vi "RFConfig_SubVI_HMCT22##_PowerOnOff.vi"(8 "error in (no error)":errorcluster, 9 "Power On?":bool, 10 "Boolean in":bool, 11 "VISA Refnum in":refnum<visa-resource-name>) -> (0 "error out":errorcluster, 3 "Boolean out":bool)   [LabVIEW 2019]
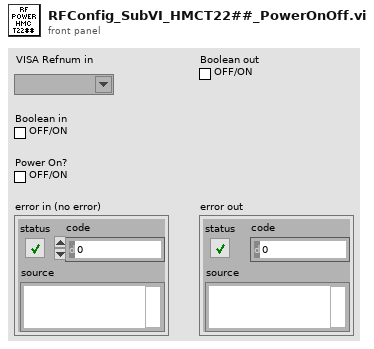
[diagram p1: front panel]
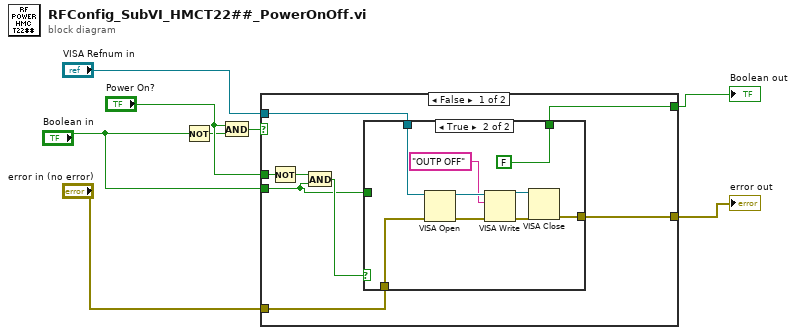
[diagram p0: block diagram]
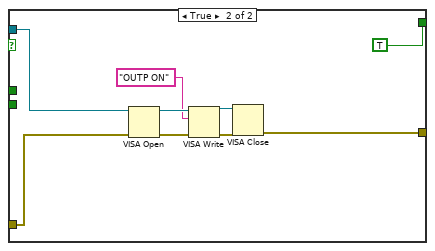
[diagram p3: hidden frame]
diagram:
  n1 = Not(x="Boolean in") -> (.not. x?=w4:bool)
  n2 = And(x="Power On?", y=w4) -> (x .and. y?=w1:bool)
  n3 = case shown="False" w1 {
    tunnel: [w11 w29] -> w2
    tunnel: "error in (no error)" -> [w12 w35]
    tunnel: "Power On?" -> [w15 _]
    tunnel: "Boolean in" -> [w9 _]
    tunnel: "VISA Refnum in" -> [w13 w36]
    tunnel: [w10 TRUE] -> w7
    frame False {
      n4 = Not(x=w15) -> (.not. x?=w16:bool)
      n5 = And(x=w16, y=w9) -> (x .and. y?=w14:bool)
      n6 = case shown="True" w14 {
        tunnel: w13 -> [_ w22]
        tunnel: w12 -> [w18 w21]
        tunnel: [w18 w20] -> w11
        tunnel: [w17 FALSE] -> w10
        tunnel: w9 -> [w17 _]
        frame False {
        }
        frame True {
          n7 = VISA Open(error in (no error)=w21, VISA resource name=w22) -> (VISA resource name=w27:refnum<visa-resource-name>, error out=w26:errorcluster)  [unwired: 3 in]
          n8 = VISA Write(VISA resource name=w27, write buffer="OUTP OFF", error in (no error)=w26) -> (VISA resource name out=w23:refnum<visa-resource-name>, error out=w24:errorcluster)  [unwired: 1 out]
          n9 = VISA Close(VISA resource name=w23, error in (no error)=w24) -> (error out=w20:errorcluster)
        }
      }
    }
    frame True {
      n10 = VISA Open(error in (no error)=w35, VISA resource name=w36) -> (VISA resource name=w34:refnum<visa-resource-name>, error out=w33:errorcluster)  [unwired: 3 in]
      n11 = VISA Write(VISA resource name=w34, write buffer="OUTP ON", error in (no error)=w33) -> (VISA resource name out=w30:refnum<visa-resource-name>, error out=w31:errorcluster)  [unwired: 1 out]
      n12 = VISA Close(VISA resource name=w30, error in (no error)=w31) -> (error out=w29:errorcluster)
    }
  }
  "Boolean out" <- w7
  "error out" <- w2
